vi "FormulaNode.vi"() -> ()   [LabVIEW 2020]
panel:
  in  "r":dbl
  out "z":dbl
  in  "y":dbl
  in  "x":dbl
  out "C":dbl
  in  "b":dbl
  in  "a":dbl
  in  "Stop Button":bool
  # "3x+5xy+8ry=z"
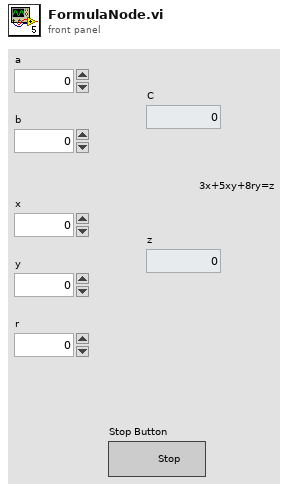
[diagram p1: front panel]
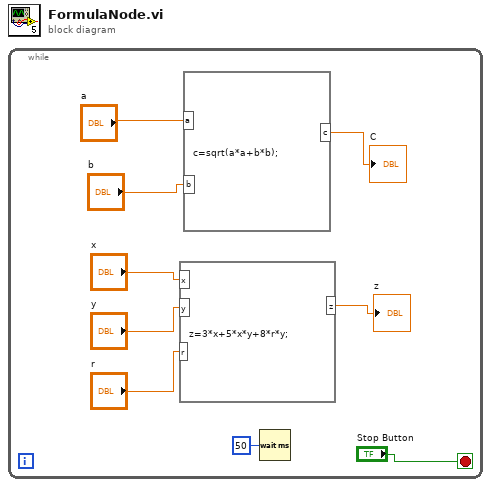
[diagram p0: block diagram]
diagram:
  n1 = while {
    stop <- "Stop Button" stop-if-true
    n2 = formula code="z=3*x+5*x*y+8*r*y;"("x"="x", "y"="y", "r"="r") -> ("z"=→"z":dbl)
    n3 = formula code="c=sqrt(a*a+b*b);"("a"="a", "b"="b") -> ("c"=→"C":dbl)
    n4 = Wait (ms)(milliseconds to wait=u32 50) -> ()  [unwired: 1 out]
  }
